vi "PH_ForceSensor.constructor.vi"(0 "name":string, 2 "data in":string, 5 "error in(no error)":errorcluster) -> (14 "i ref out":refnum<vi>, 16 "data out":string, 19 "error out":errorcluster)   [LabVIEW 2014, in "PH_ForceSensor.lvlib"]
doc: "This class is forseen to control black boxes (motion).\n\nThis class is part of the PHELIX device layer.\n\nauthor: Stefan Götte, GSI\n\nLicense Agreement for this software:\n\nCopyright (C)\nGesellschaft für Schwerionenforschung, GSI\nPlanckstr. 1\n64291 Darmstadt\nGermany\n\nContact: D.Beck@gsi.de \n\nThis program is free software; you can redistribute it and/or modify it under the terms of the \nGNU General Public License as published by the Free Software Foundation; either version 2 of \nthe license, or (at your option) any later version.\n\nThis program is distributed in the hope that it will be useful, but WITHOUT ANY WARRANTY; \nwithout even the implied warranty of MERCHANTABILITY or FITNESS FOR A PARTICULAR PURPOSE. See the GNU General License for more details (http://www.gnu.org).\n\nGesellschaft für Schwerionenforschung, GSI\nPlanckstr. 1, 64291 Darmstadt, Germany\nFor all questions and ideas contact: M.Richter@gsi.de, H.Brand@gsi.de or D.Beck@gsi.de.\nLast update: 16-JUN-2004"
uses:
  PH_ForceSensor.lvlib
  PH_Basics/PH_Class/PH_Class.lvlib
  CS_Core/CSSystem/CSSystemLib/CSSystemLib.lvlib
  PH_Basics/PH_PSDBWriter/PH_PSDBWriter.lvlib
  PHELIX/PH_BeamlineInformation/PH_BeamlineInformation.lvlib
  PH_Basics/PH_StatusHandler/PH_StatusHandler.lvlib
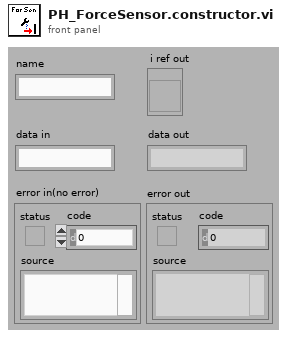
[diagram p1: front panel]
types:
  T1 = enum16{"SetAttribute", "GetAttribute", "CreateAttribute", "DestroyAttribute", "DestroyAllAtributes"}
  T2 = typedef "PH_ForceSensor.lvlib/PH_ForceSensor.i attribute.ctl" = cluster{"GUI Refs":T3, "Rawvalues":T4, "Offsets [µV]":T4, "Scalings [mV/V]":T4, "Forces [N]":T4, "Supply Voltage [V]":dbl, "Full Force [N]":dbl, "Ranges [N]":cluster{"Low Energy":cluster{"Upper Limit":dbl, "Lower Limit":dbl}, "High Energy":cluster{"Upper Limit":dbl, "Lower Limit":dbl}}}
  T3 = typedef "PH_ForceSensor.lvlib/PH_ForceSensor.GUI Refs.ctl" = cluster{"Delete":refnum<vi>, "Rawvalues":refnum<vi>, "Offsets [µV]":refnum<vi>, "Sensor Values [µV]":refnum<vi>, "Scalings [mV/V]":refnum<vi>, "Supply Voltage [V]":refnum<vi>, "Full Force [N]":refnum<vi>, "Forces [N]":refnum<vi>, "Graph Differential Forces":refnum<vi>, "Graph Absolute Forces":refnum<vi>, "Ranges [N]":refnum<vi>}
  T4 = typedef "PH_ForceSensor.lvlib/PH_ForceSensor.Dataset.ctl" = cluster{"top front":dbl, "top back":dbl, "bottom front":dbl, "bottom back":dbl}
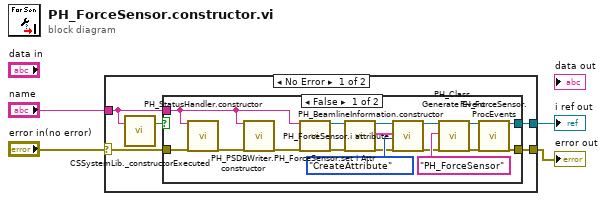
[diagram p0: block diagram]
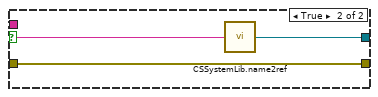
[diagram p2: hidden frame]
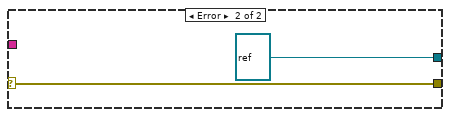
[diagram p3: hidden frame]
diagram:
  n1 = case shown="No Error" "error in(no error)" {
    selector: "error in(no error)" -> [w9 w31]
    tunnel: [w8 refnum<vi> refnum ("i ref out")] -> w4
    tunnel: [w7 w31] -> w3
    tunnel: "name" -> [w6 _]
    frame No Error {
      n2 = call "CSSystemLib._constructorExecuted.vi"("name"=w6) -> ("constructor executed?"=w5:bool)  [unwired: 18 in]
      n3 = case shown="False" w5 {
        tunnel: w9 -> [w16 w29]
        tunnel: [w22 w27] -> w8
        tunnel: [w21 w29] -> w7
        tunnel: w6 -> [w10 w28]
        frame False {
          n4 = call "PH_StatusHandler.constructor.vi"("name"=w10, "error in(no error)"=w16) -> ("error out"=w11:errorcluster)  [unwired: 15 in, 2 out]
          n5 = call "PH_PSDBWriter.constructor.vi"("name"=w10, "error in"=w11) -> ("error out"=w19:errorcluster)  [unwired: 15 in, 2 out]
          n6 = call "PH_BeamlineInformation.constructor.vi"("name"=w10, "error in(no error)"=w19) -> ("i ref out"=w12:refnum<vi>, "error out"=w13:errorcluster)  [unwired: 15 in, 1 out]
          n7 = call "PH_ForceSensor.set i Attr.vi"("VI in"=w12, "error in (no error)"=w13) -> ("VI out"=w24:refnum<vi>, "i Attribute"=w25:T2, "error out"=w23:errorcluster)  [unwired: 15 in]
          n8 = call "PH_ForceSensor.i attribute.vi"("VI Refnum"=w24, "CLASS.i attribute"=w25, "Action"=T1."CreateAttribute", "error in (no error)"=w23) -> ("VI Refnum out"=w18:refnum<vi>, "error out"=w17:errorcluster)  [unwired: 13 in, 1 out]
          n9 = call "PH_Class.Generate Event.vi"("i ref in"=w18, "Class"="PH_ForceSensor", "error in (no error)"=w17) -> ("i ref out"=w15:refnum<vi>, "error out"=w14:errorcluster)  [unwired: 15 in]
          n10 = call "PH_ForceSensor.ProcEvents.vi"("i ref in"=w15, "error in (no error)"=w14) -> ("i ref out"=w22:refnum<vi>, "error out"=w21:errorcluster)  [unwired: 16 in]
        }
        frame True {
          n11 = call "CSSystemLib.name2ref.vi"("name"=w28) -> ("obj refnum"=w27:refnum<vi>)
        }
      }
    }
    frame Error {
    }
  }
  "i ref out" <- w4
  "error out" <- w3
